vi "Control_Source_Valve.vi"(0 "Source Valve":bool) -> (1 "Error Comments":string, 2 "Voltage Set":dbl format="%.2f")   [LabVIEW 2010]
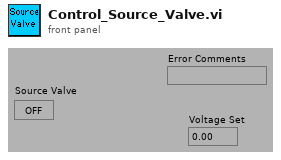
[diagram p1: front panel]
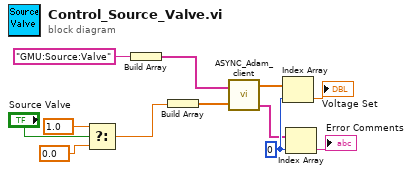
[diagram p0: block diagram]
diagram:
  w12 = 0 ("Index")
  n1 = Select(t=1.0, s="Source Valve", f=0.0) -> (s? t:f=w1:dbl)
  n2 = Build Array("GMU:Source:Valve") -> (w8:string[])
  n3 = Build Array(w1) -> (w9:dbl[])
  n4 = call "ASYNC_Adam_client.vi"("Values"=w9, "Channel Names"=w8) -> ("Scan Comments"=w11:string[], "Calibrated Units"=w10:dbl[])
  n5 = Index Array(array=w10, index=w12) -> (element=→"Voltage Set":dbl)
  n6 = Index Array(array=w11, index=w12) -> (element=→"Error Comments":string)
